vi "Teleop.vi"(10 "Match Info":T1={"Autonomous Elapsed Seconds"=0.0, "TeleOp Elapsed Seconds"=0.0, "Disabled Elapsed Seconds"=0.0, "Visited Autonomous"=FALSE, "Visited TeleOp"=FALSE, "Visited Disabled"=FALSE, "Autonomous Settings"={"Autonomous Style"=enum."Independent", "VI Refnum"=refnum}}, 11 "Call Context":T2) -> ()   [LabVIEW 2015]
doc: "This VI is called for each TeleOp packet received from the DS where the robot is not disabled. It is often used to read from the joysticks and update I/O or to update setpoints for timed control loops. It should complete and return within 20 milliseconds or it may miss DS packets."
uses:
  <vilib>/Rock Robotics/WPI/DriverStation/WPI_DriverStationDerivedRobotMode.ctl
  <vilib>/Rock Robotics/WPI/DriverStation/WPI_DriverStationMatch Info.ctl
  <vilib>/Rock Robotics/WPI/Relay/WPI_RelayValue.ctl
  <vilib>/Rock Robotics/WPI/Utilities/WPI_GetSetVariantRefNum.vi
  <vilib>/Rock Robotics/Network Tables/NT Write Boolean Array.vi
  <vilib>/Rock Robotics/Network Tables/NT Write Numeric Array.vi
  <vilib>/Rock Robotics/Network Tables/NT Read Boolean.vi
  <vilib>/Rock Robotics/Network Tables/NT Read Number.vi
panel:
  out "Sample Slider 0":dbl(slide) scale=0.0..5.0
  out "Sample Boolean 1":bool
  out "Sample Boolean 0":bool
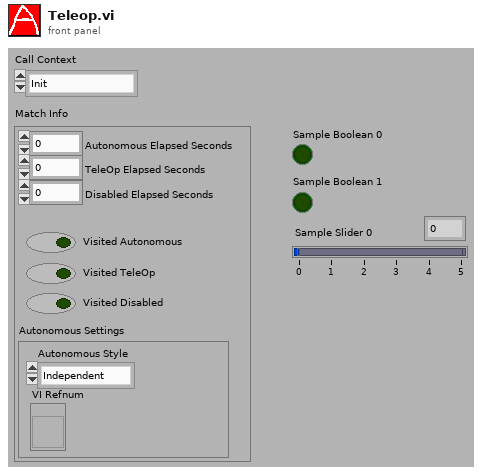
[diagram p1: front panel]
types:
  T1 = typedef "WPI_DriverStationMatch Info.ctl" = cluster{"Autonomous Elapsed Seconds":dbl, "TeleOp Elapsed Seconds":dbl, "Disabled Elapsed Seconds":dbl, "Visited Autonomous":bool, "Visited TeleOp":bool, "Visited Disabled":bool, "Autonomous Settings":cluster{"Autonomous Style":enum16{"Iterative", "Independent"}, "VI Refnum":refnum<vi>}}
  T2 = typedef "WPI_DriverStationDerivedRobotMode.ctl" = enum16{"Init", "Execute", "Stop"}
  T3 = typedef "WPI_JoystickDevRef.ctl" = cluster{"Device":T4}
  T4 = typedef "WPI_JoystickDeviceEnum.ctl" = enum16{"USB 0", "USB 1", "USB 2", "USB 3", "USB 4", "USB 5"}
  T5 = typedef "WPI_RelayValue.ctl" = enum16{"Off", "On", "Forward", "Reverse"}
  T6 = typedef "WPI_RelayDevRef.ctl" = cluster{"DevStatus":errorcluster, "Relay Channel":T7, "Relay Direction":T8}
  T7 = typedef "FPGA_DIORelayChannel.ctl" = enum8{"Relay 0", "Relay 1", "Relay 2", "Relay 3", "Invalid"}
  T8 = typedef "WPI_RelayDirection.ctl" = enum16{"Both directions", "Forward only", "Reverse only"}
  T9 = typedef "WPI_MotorControlDeviceRef.ctl" = cluster{"DeviceStatus":errorcluster, "Type":T10, "PWM":cluster{"PWM Channel":T11, "DeadBand":T12}, "CAN":cluster{"Device Number":u8, "Control Mode":T13, "Semaphore":T14, "Max Vout":dbl, "TalonSRX Control Mode":T15}, "Invert":bool}
  T10 = typedef "WPI_MotorControlType.ctl" = enum16{"PWM", "CAN", "CANTalonSRX"}
  T11 = typedef "FPGA_DIOPWMChannel.ctl" = enum8{"PWM 0", "PWM 1", "PWM 2", "PWM 3", "PWM 4", "PWM 5", "PWM 6", "PWM 7", "PWM 8", "PWM 9", "PWM MXP 0", "PWM MXP 1", "PWM MXP 2", "PWM MXP 3", "PWM MXP 4", "PWM MXP 5", "PWM MXP 6", "PWM MXP 7", "PWM MXP 8", "PWM MXP 9", "Invalid"}
  T12 = typedef "WPI_PWMDeadband.ctl" = cluster{"Name":string, "maxPositivePwm":i32, "minPositivePwm":i32, "centerPwm":i32, "maxNegativePwm":i32, "minNegativePwm":i32, "angularRange":u16}
  T13 = typedef "WPI_CANJaguar_ControlMode.ctl" = enum8{"Percent VBus", "Current", "Speed", "Position", "Voltage"}
  T14 = typedef "Semaphore RefNum" = refnum<k1>
  T15 = typedef "WPI_CANTalonSRX_APIControlMode.ctl" = enum8{"Percent VBus", "Speed", "Position", "Slave", "Unchanged / Invalid", "Voltage Compensation", "Current", "Motion Profile"}
  T16 = typedef "WPI_RobotDriveDevRef.ctl" = cluster{"DevStatus":errorcluster, "Motors[]":T9[], "Square Inputs":bool, "Max Output":dbl}
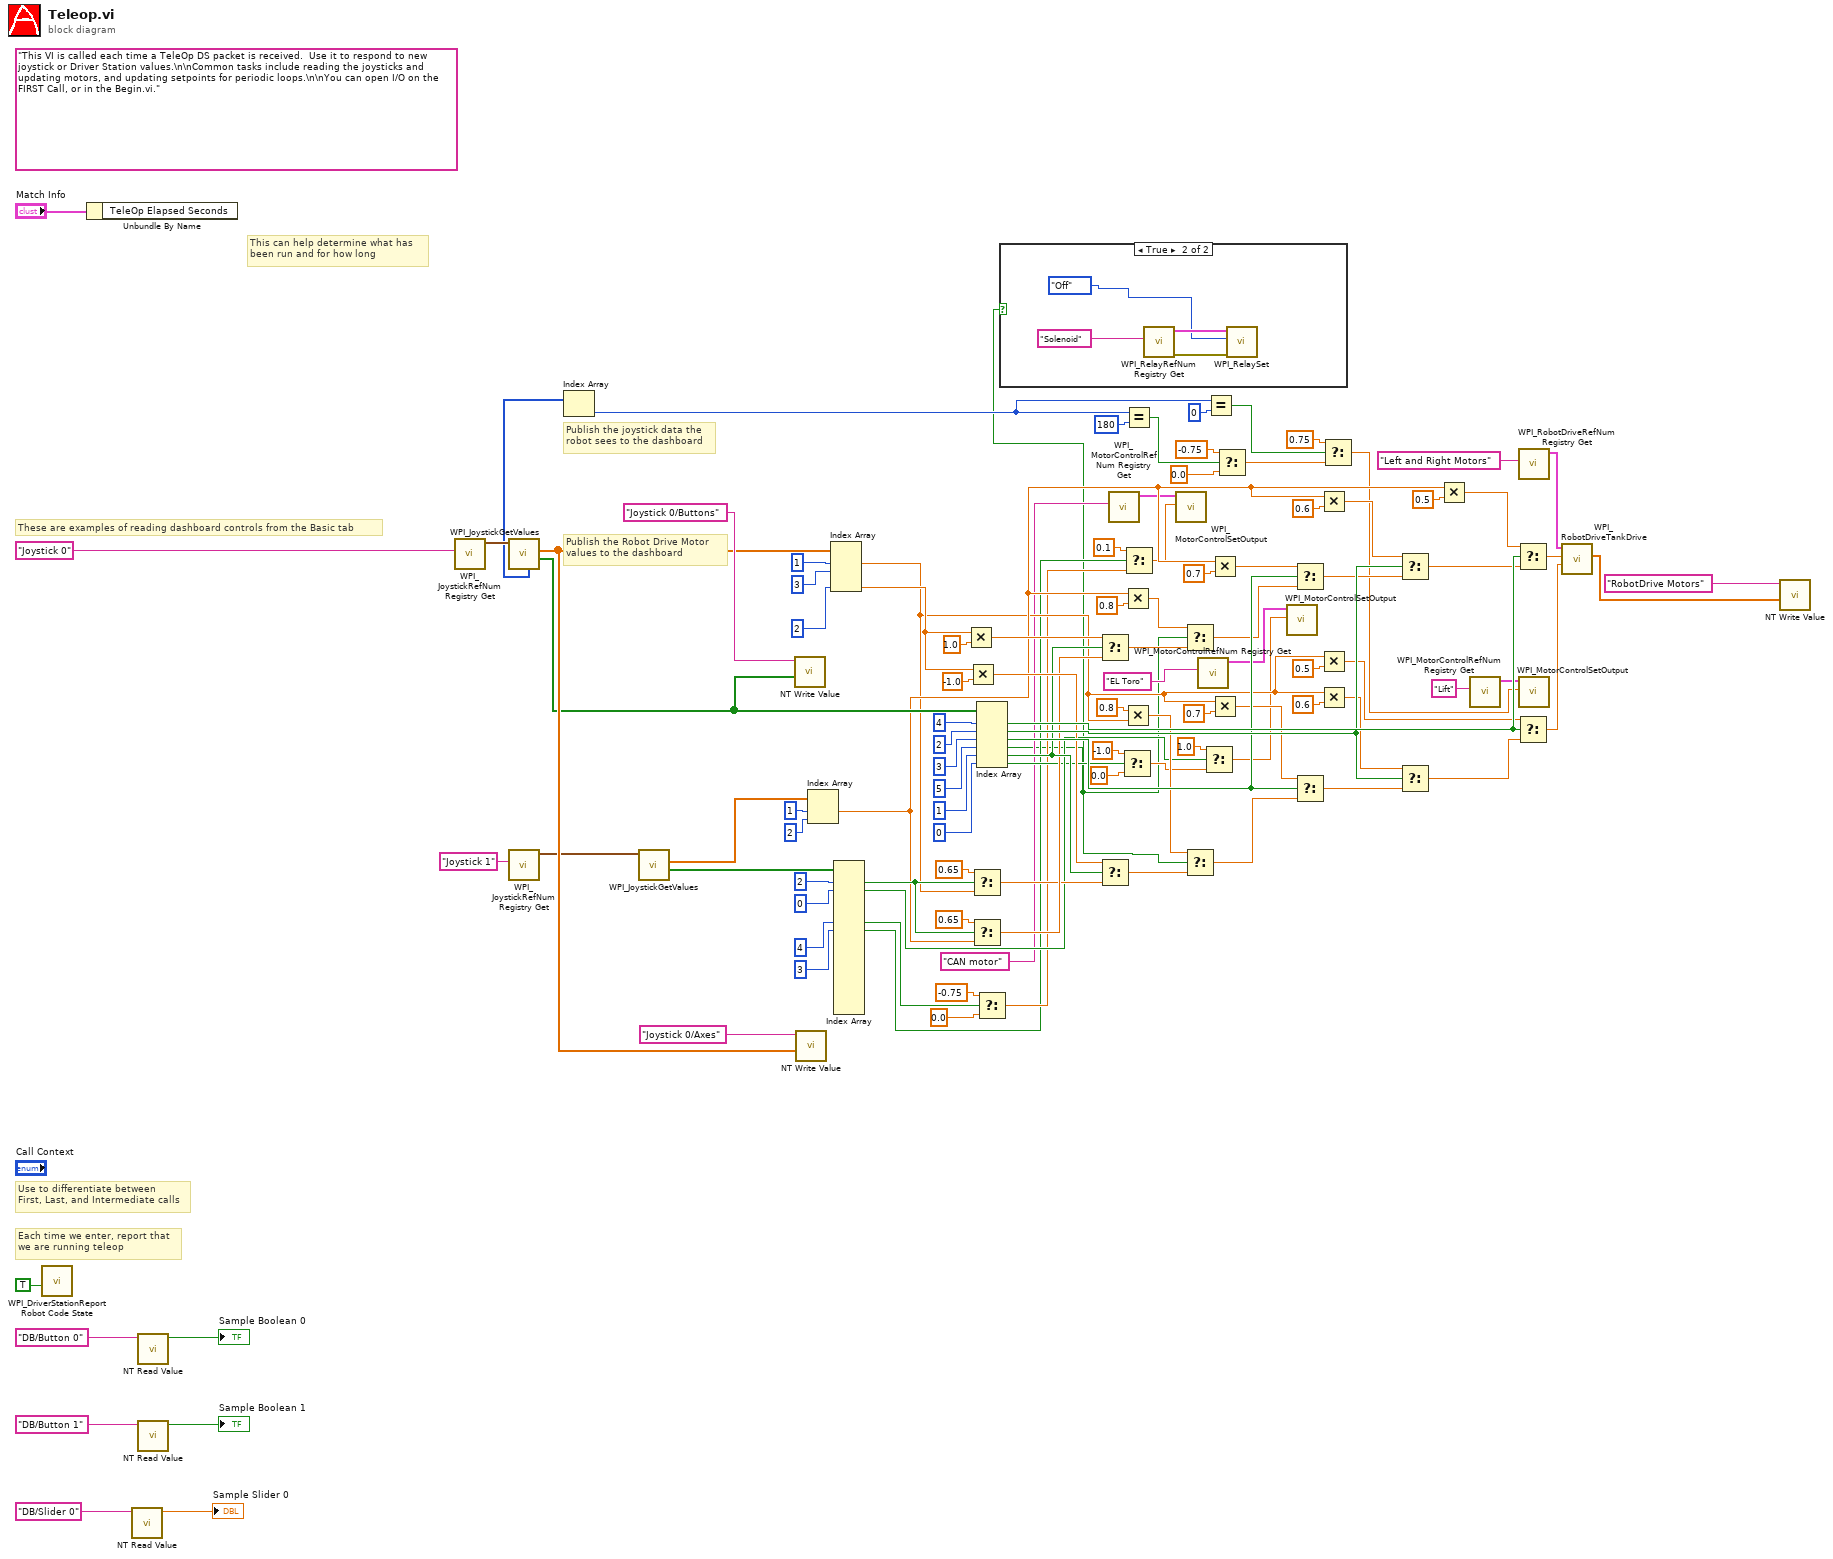
[diagram p0: block diagram]
diagram:
  (unwired) "This VI is called each time a TeleOp DS packet is received.  Use it to respond to new joystick or Driver Station values.\n\nCommon tasks include reading the joysticks and updating motors, and updating setpoints for periodic loops.\n\nYou can open I/O on the FIRST Call, or in the Begin.vi."
  # "These are examples of reading dashboard controls from the Basic tab"
  # "Publish the Robot Drive Motor\nvalues to the dashboard"
  # "Publish the joystick data the\nrobot sees to the dashboard"
  # "Each time we enter, report that\nwe are running teleop"
  # "Use to differentiate between\nFirst, Last, and Intermediate calls"
  # "This can help determine what has\nbeen run and for how long"
  n1 = call <vilib>:"WPI_DriverStationReport Robot Code State.vi"("TeleOp"=TRUE ("Autonomous")) -> ()  [unwired: 10 in, 1 out]
  n2 = Unbundle By Name("Match Info") -> ()  [unwired: 1 out]
  n3 = call-poly <vilib>:"NT Read Value.vi"("Name"="DB/Slider 0" ("refnum name")) -> ("Numeric"=→"Sample Slider 0":dbl)  [unwired: 9 in, 1 out]
  n4 = call-poly <vilib>:"NT Read Value.vi"("Name"="DB/Button 0" ("refnum name")) -> ("Boolean"=→"Sample Boolean 0":bool)  [unwired: 9 in, 1 out]
  n5 = call-poly <vilib>:"NT Read Value.vi"("Name"="DB/Button 1" ("refnum name")) -> ("Boolean"=→"Sample Boolean 1":bool)  [unwired: 9 in, 1 out]
  n6 = call <vilib>:"WPI_JoystickRefNum Registry Get.vi"("refnum name"="Joystick 0") -> ("JoystickDevRef"=w108:T3)  [unwired: 1 in, 9 out]
  n7 = call <vilib>:"WPI_JoystickGetValues.vi"("JoystickDevRef"=w108) -> ("Buttons"=w56:bool[], "Axes"=w104:dbl[], "POVs"=w18:i16[])  [unwired: 6 in, 2 out]
  n8 = call <vilib>:"WPI_JoystickRefNum Registry Get.vi"("refnum name"="Joystick 1") -> ("JoystickDevRef"=w94:T3)  [unwired: 1 in, 9 out]
  n9 = Index Array(array=w18) -> (element=w17:i16)  [unwired: 1 in]
  n10 = call <vilib>:"WPI_JoystickGetValues.vi"("JoystickDevRef"=w94) -> ("Buttons"=w55:bool[], "Axes"=w92:dbl[])  [unwired: 6 in, 3 out]
  n11 = call-poly <vilib>:"NT Write Value.vi"("Boolean Array"=w56, "Name"="Joystick 0/Buttons") -> ()  [unwired: 9 in, 1 out]
  n12 = call-poly <vilib>:"NT Write Value.vi"("Numeric Array"=w104, "Name"="Joystick 0/Axes") -> ()  [unwired: 9 in, 1 out]
  n13 = Index Array(array=w92, index #1=1 ("index"), index #2=2 ("index")) -> (element #1=w39:dbl)  [unwired: 1 out]
  n14 = Index Array(array=w104, index #1=1 ("index"), index #2=3 ("index"), index #4=2 ("index")) -> (element #1=w37:dbl, element #4=w54:dbl)  [unwired: 1 in, 2 out]
  n15 = Index Array(array=w55, index #1=2 ("index"), index #2=0 ("index"), index #6=4 ("index"), index #7=3 ("index")) -> (element #1=w42:bool, element #2=w22:bool, element #6=w5:bool, element #7=w4:bool)  [unwired: 13 in, 13 out]
  n16 = Multiply(x=w54, y=1.0) -> (x*y=w52:dbl)
  n17 = Multiply(x=w54, y=-1.0) -> (x*y=w53:dbl)
  n18 = Select(t=0.65, s=w42, f=w37) -> (s? t:f=w38:dbl)
  n19 = Select(t=0.65, s=w42, f=w39) -> (s? t:f=w40:dbl)
  n20 = Index Array(array=w56, index #1=4 ("index"), index #2=2 ("index"), index #3=3 ("index"), index #4=5 ("index"), index #5=1 ("index"), index #6=0 ("index")) -> (element #1=w85:bool, element #2=w84:bool, element #3=w83:bool, element #4=w1:bool, element #5=w47:bool, element #6=w19:bool)
  n21 = Select(t=-0.75, s=w5, f=0.0) -> (s? t:f=w8:dbl)
  n22 = case shown="True" w1 {
    frame False {
    }
    frame True {
      n23 = call <vilib>:"WPI_RelayRefNum Registry Get.vi"("refnum name"="Solenoid") -> ("error out"=w114:errorcluster, "RelayDevRef"=w113:T6)  [unwired: 9 in]
      n24 = call <vilib>:"WPI_RelaySet.vi"("error in (no error)"=w114, "RelayValue"=WPI_RelayValue."Off", "RelayDevRef"=w113) -> ()  [unwired: 7 in, 2 out]
    }
  }
  n25 = Select(t=w52, s=w47, f=w40) -> (s? t:f=w48:dbl)
  n26 = Select(t=w53, s=w47, f=w38) -> (s? t:f=w49:dbl)
  n27 = call <vilib>:"WPI_MotorControlRefNum Registry Get.vi"("refnum name"="CAN motor") -> ("MotorControlDevRef"=w15:T9)  [unwired: 9 in, 1 out]
  n28 = Select(t=-1.0, s=w19, f=0.0) -> (s? t:f=w32:dbl)
  n29 = Multiply(x=w39, y=0.8 ("t")) -> (x*y=w58:dbl)
  n30 = Multiply(x=0.8 ("t"), y=w37) -> (x*y=w57:dbl)
  n31 = Equal?(x=w17, y=i16 180) -> (x = y?=w2:bool)
  n32 = Select(t=0.1, s=w4, f=w8) -> (s? t:f=w7:dbl)
  n33 = call <vilib>:"WPI_MotorControlSetOutput.vi"("Output"=w7, "MotorControlDevRef"=w15) -> ()  [unwired: 7 in, 3 out]
  n34 = Select(t=w58, s=w1, f=w48) -> (s? t:f=w68:dbl)
  n35 = Select(t=w57, s=w1, f=w49) -> (s? t:f=w75:dbl)
  n36 = call <vilib>:"WPI_MotorControlRefNum Registry Get.vi"("refnum name"="EL Toro") -> ("MotorControlDevRef"=w35:T9)  [unwired: 9 in, 1 out]
  n37 = Select(t=1.0, s=w22, f=w32) -> (s? t:f=w31:dbl)
  n38 = Equal?(x=w17, y=i16 0) -> (x = y?=w29:bool)
  n39 = Multiply(x=w39, y=0.7 ("t")) -> (x*y=w67:dbl)
  n40 = Multiply(x=w37, y=0.7 ("t")) -> (x*y=w74:dbl)
  n41 = Select(t=-0.75, s=w2, f=0.0) -> (s? t:f=w26:dbl)
  n42 = call <vilib>:"WPI_MotorControlSetOutput.vi"("Output"=w31, "MotorControlDevRef"=w35) -> ()  [unwired: 7 in, 3 out]
  n43 = Select(t=w67, s=w83, f=w68) -> (s? t:f=w69:dbl)
  n44 = Select(t=w74, s=w83, f=w75) -> (s? t:f=w76:dbl)
  n45 = Multiply(x=w39, y=0.6 ("t")) -> (x*y=w65:dbl)
  n46 = Multiply(x=w37, y=0.5) -> (x*y=w78:dbl)
  n47 = Multiply(x=w37, y=0.6 ("t")) -> (x*y=w72:dbl)
  n48 = Select(t=0.75, s=w29, f=w26) -> (s? t:f=w13:dbl)
  n49 = Select(t=w65, s=w84, f=w69) -> (s? t:f=w63:dbl)
  n50 = Select(t=w72, s=w84, f=w76) -> (s? t:f=w77:dbl)
  n51 = Multiply(x=w39, y=0.5) -> (x*y=w62:dbl)
  n52 = call <vilib>:"WPI_MotorControlRefNum Registry Get.vi"("refnum name"="Lift") -> ("MotorControlDevRef"=w11:T9)  [unwired: 9 in, 1 out]
  n53 = Select(t=w62, s=w85, f=w63) -> (s? t:f=w81:dbl)
  n54 = Select(t=w78, s=w85, f=w77) -> (s? t:f=w82:dbl)
  n55 = call <vilib>:"WPI_RobotDriveRefNum Registry Get.vi"("refnum name"="Left and Right Motors") -> ("RobotDriveDevRef"=w95:T16)  [unwired: 1 in, 9 out]
  n56 = call <vilib>:"WPI_MotorControlSetOutput.vi"("Output"=w13, "MotorControlDevRef"=w11) -> ()  [unwired: 7 in, 3 out]
  n57 = call <vilib>:"WPI_RobotDriveTankDrive.vi"("Right axis value"=w82, "Left axis value"=w81, "RobotDriveDevRef"=w95) -> ("Motor Values"=w96:dbl[])  [unwired: 6 in, 2 out]
  n58 = call-poly <vilib>:"NT Write Value.vi"("Numeric Array"=w96, "Name"="RobotDrive Motors") -> ()  [unwired: 9 in, 1 out]
